vi "_FPGA_ConjSelector_rev2.vi"(0 "Conj.InitCyc*2^32":u32, 1 "ConjArr":T1(array[cluster])=[{"Len"=0, "CycleDiff"=0, "Times"=0}, {"Len"=0, "CycleDiff"=0, "Times"=0}, {"Len"=0, "CycleDiff"=0, "Times"=0}, {"Len"=0, "CycleDiff"=0, "Times"=0}, {"Len"=0, "CycleDiff"=0, "Times"=0}, {"Len"=0, "CycleDiff"=0, "Times"=0}, {"Len"=0, "CycleDiff"=0, "Times"=0}, {"Len"=0, "CycleDiff"=0, "Times"=0}], 2 "Init_strobe":bool, 5 "ConjSize-1":u8, 11 "RfNxtCyc_in":u64) -> (3 "LastConj":bool, 4 "ConjIndex":u8, 6 "Initialising?":bool, 10 "Not Conj?":bool, 14 "Cross Conj?":bool)   [LabVIEW 2018]
uses:
  <instrlib>/_niInstr/Basic Elements/v1/FPGA/Private/Count Down U16.vi
  <instrlib>/_niInstr/Basic Elements/v1/FPGA/Private/Count Down U8.vi
  <instrlib>/_niInstr/Basic Elements/v1/FPGA/niInstr Basic Elements v1 FPGA.lvlib
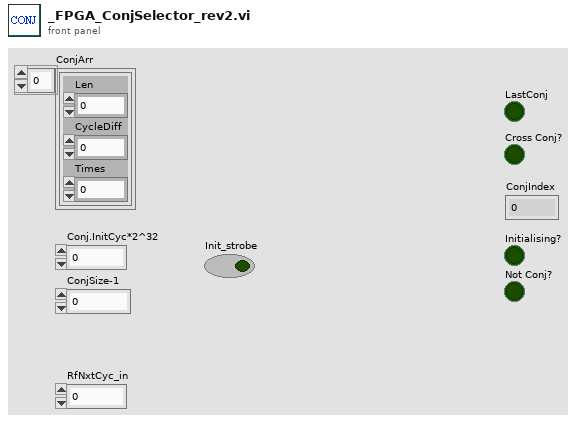
[diagram p1: front panel]
types:
  T1 = cluster{"Len":u16, "CycleDiff":u64, "Times":u8}[]
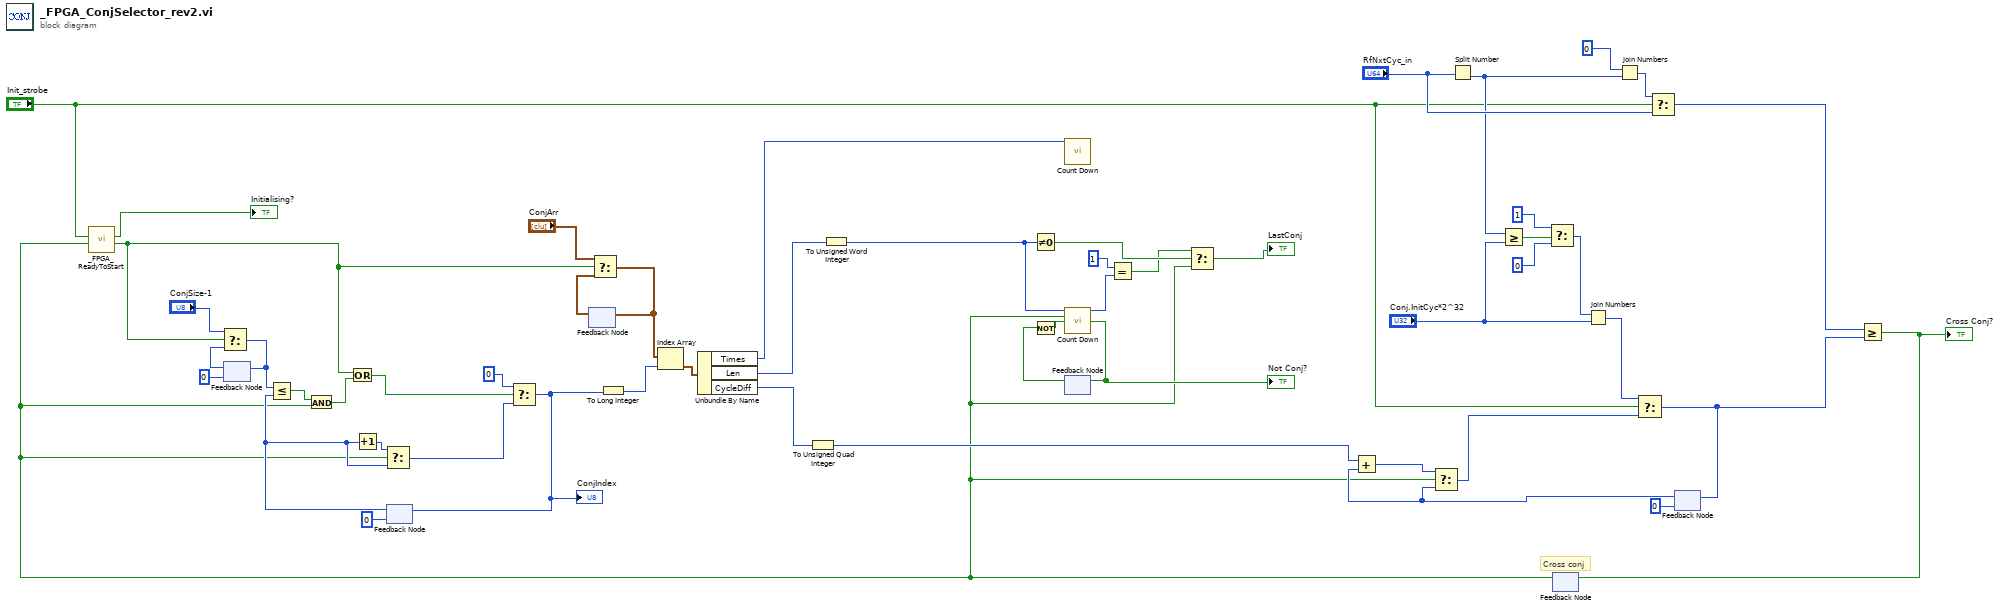
[diagram p0: block diagram]
diagram:
  # "Cross conj"
  n1 = feedback #1(u8 0 ("ConjSize-1")) -> (w30:u8)
  n2 = feedback #2(u8 0) -> (w47:u8)
  n3 = Increment(x=w47) -> (x+1=w48:u8)
  n4 = feedback #3() -> (w43:T1)  [unwired: 1 in]
  n5 = feedback #4() -> (w33:bool)  [unwired: 1 in]
  n6 = Not(x=w33) -> (.not. x?=w34:bool)
  n7 = Split Number(x="RfNxtCyc_in") -> (lo(x)=w26:u32)  [unwired: 1 out]
  n8 = Greater Or Equal?(x=w26, y="Conj.InitCyc*2^32") -> (x >= y?=w24:bool)
  n9 = Select(t=u32 1 ("hi"), s=w24, f=u32 0 ("hi(x)")) -> (s? t:f=w21:u32)
  n10 = feedback #5() -> (w8:bool)  [unwired: 1 in]
  n11 = call "_FPGA_ReadyToStart.vi"("Start_strobe_in"=w8, "Ready_latch_in"="Init_strobe") -> ("Trigger_strobe_out"=w6:bool, "Ready?"=→"Initialising?":bool)  [unwired: 8 in]
  n12 = Select(t="ConjSize-1", s=w6, f=w30) -> (s? t:f=w31:u8)
  n13 = feedback-in #1(w31) -> ()
  n14 = Less Or Equal?(x=w31, y=w47) -> (x <= y?=w50:bool)
  n15 = And(x=w50, y=w8) -> (x .and. y?=w36:bool)
  n16 = Or(x=w6, y=w36) -> (x .or. y?=w28:bool)
  n17 = Select(t=w48, s=w8, f=w47) -> (s? t:f=w45:u8)
  n18 = Select(t=u8 0, s=w28, f=w45) -> (s? t:f=w37:u8)
  "ConjIndex" <- w37
  n19 = feedback-in #2(w37) -> ()
  n20 = Select(t="ConjArr", s=w6, f=w43) -> (s? t:f=w35:T1)
  n21 = feedback-in #3(w35) -> ()
  n22 = To Long Integer(number=w37) -> (32bit integer=w51:i32)
  n23 = Index Array(array=w35, index=w51) -> (element=w52:cluster{"Len":u16, "CycleDiff":u64, "Times":u8})
  n24 = Unbundle By Name(w52) -> ("Times"=w1:u8, "Len"=w2:u16, "CycleDiff"=w3:u64)
  n25 = To Unsigned Quad Integer(1:w3) -> (0:w29:u64)
  n26 = To Unsigned Word Integer(number=w2) -> (unsigned 16bit integer=w4:u16)
  n27 = Not Equal To 0?(x=w4) -> (x != 0?=w12:bool)
  n28 = call-poly <instrlib>:"Count Down.vi"("count in"=w1) -> ()  [unwired: 13 in, 2 out]
  n29 = call-poly <instrlib>:"Count Down.vi"("count in"=w4, "load"=w8, "decrement"=w34) -> ("count out"=w14:u16, "terminal count"=w9:bool)  [unwired: 11 in]
  "Not Conj?" <- w9
  n30 = feedback-in #4(w9) -> ()
  n31 = Equal?(x=u16 1, y=w14) -> (x = y?=w11:bool)
  n32 = Select(t=w11, s=w12, f=w8) -> (s? t:f=→"LastConj":bool)
  n33 = Join Numbers(hi=w21, lo="Conj.InitCyc*2^32") -> ((hi.lo)=w20:u64)
  n34 = Join Numbers(hi=u32 0 ("hi(x)"), lo=w26) -> ((hi.lo)=w40:u64)
  n35 = Select(t=w40, s="Init_strobe", f="RfNxtCyc_in") -> (s? t:f=w19:u64)
  n36 = feedback #6(u64 0) -> (w44:u64)
  n37 = Add(x=w29, y=w44) -> (x+y=w49:u64)
  n38 = Select(t=w49, s=w8, f=w44) -> (s? t:f=w42:u64)
  n39 = Select(t=w20, s="Init_strobe", f=w42) -> (s? t:f=w39:u64)
  n40 = feedback-in #6(w39) -> ()
  n41 = Greater Or Equal?(x=w19, y=w39) -> (x >= y?=w38:bool)
  "Cross Conj?" <- w38
  n42 = feedback-in #5(w38) -> ()
